vi "Guard clause.vi"(8 "error in":errorcluster, 10 "queue - error handler":refnum<queue>, 11 "queue - message":refnum<queue>) -> (0 "error out":errorcluster, 2 "message":string, 3 "queue out":refnum<queue>)   [LabVIEW 2021]
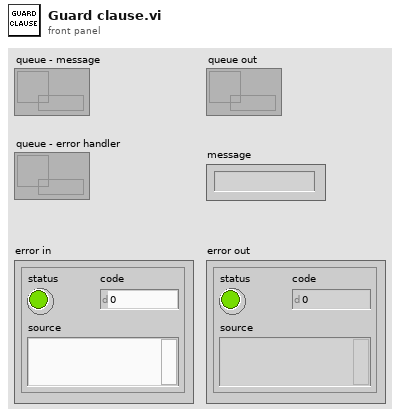
[diagram p1: front panel]
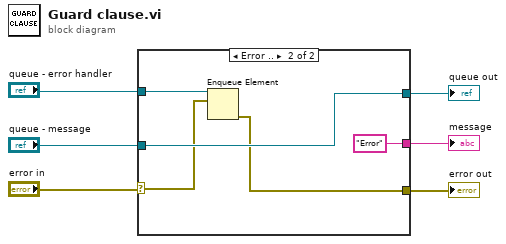
[diagram p0: block diagram]
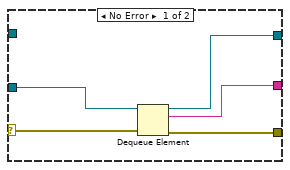
[diagram p2: hidden frame]
diagram:
  n1 = case shown="Error .." "error in" {
    selector: "error in" -> [w11 w13]
    tunnel: [w10 w14] -> w5
    tunnel: [w9 "Error"] -> w4
    tunnel: "queue - message" -> [w8 w15]
    tunnel: [w7 w15] -> w2
    tunnel: "queue - error handler" -> [_ w12]
    frame No Error {
      n2 = Dequeue Element(queue=w8, error in (no error)=w11) -> (queue out=w7:refnum<queue>, element=w9:string, error out=w10:errorcluster)  [unwired: 1 in, 1 out]
    }
    frame Error {
      n3 = Enqueue Element(queue=w12, element=w13) -> (error out=w14:errorcluster)  [unwired: 2 in, 2 out]
    }
  }
  "error out" <- w5
  "message" <- w4
  "queue out" <- w2
